vi "AuxReadThresholds.vi"() -> ()   [LabVIEW 2017]
panel:
  out "threshholds":cluster{"t1 pmt":i32, "t1 camera":i32}
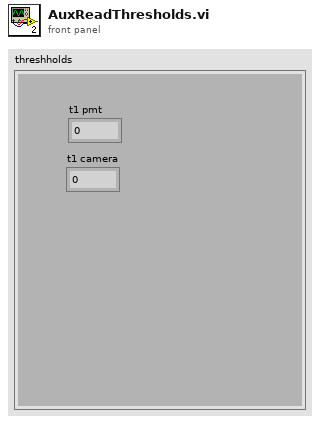
[diagram p1: front panel]
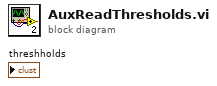
[diagram p0: block diagram]
diagram:
